vi "Initialize Core.vi"(8 "error in":errorcluster, 10 "Shared Resources":refnum<class "Shared Resources.lvclass">, 11 "Tx Acyclic Labels Execution Unit in":refnum<class "Tx Acyclic Labels Execution Unit.lvclass">) -> (0 "error out":errorcluster, 3 "Tx Acyclic Labels Execution Unit out":refnum<class "Tx Acyclic Labels Execution Unit.lvclass">)   [LabVIEW 2020, in "AIM ARINC 429 Engine.lvlib" / "Implementation.lvlib" / "Tx Acyclic Labels Execution Unit.lvclass"]
uses:
  Tx Acyclic Labels Execution Unit.lvclass
  C:/git/ni/niveristand-aim-arinc429-custom-device/Source/Custom Device Support/Engine/Implementation/Execution Unit/Execution Unit.lvclass
  Shared Resources/Shared Resources.lvclass
  Execution Unit/Execution Unit.lvclass/Execution Unit.ctl
  Tx Acyclic Labels Execution Unit.lvclass/Tx Acyclic Labels Execution Unit.ctl
  Execution Unit/Read board handle.vi
  Hardware API/AIM ARINC 429 Hardware API.lvlib
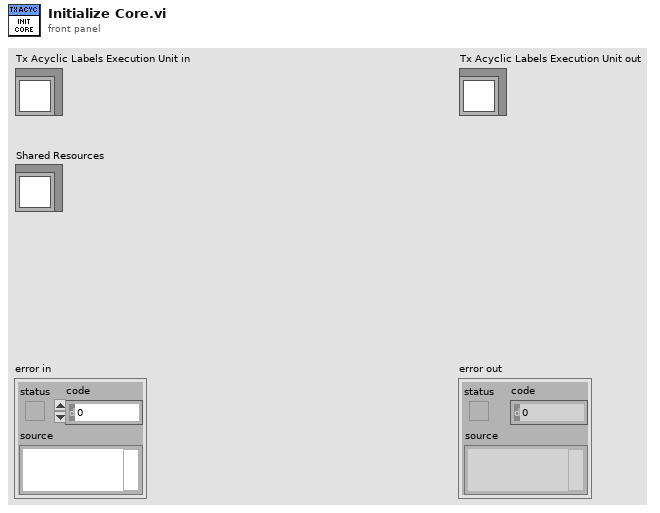
[diagram p1: front panel]
types:
  T1 = typedef "RT Hardware Channel Settings.ctl" = cluster{"channel #":u16, "channel handle":u64, "labels settings for RT":T2[], "speed":T10}
  T2 = typedef "RT Label Settings.ctl" = cluster{"Name":string, "xmlName":string, "label":T3, "transfer period":u32, "SDI_Enabled":bool, "SDI":u8, "parameter driver data":T4, "transfer type":T8, "has timestamp?":bool, "Label Disable/Trigger Channel Reference":T7, "Message Handle":u64, "Initialized?":bool, "Word Initial Raw Value":u32, "Label Timestamp Channel Data Reference":T9, "disabled":bool}
  T3 = typedef "Label.ctl" = u8
  T4 = typedef "RT Parameters.ctl" = cluster{"parameter definitions":T5[], "Tx parameter refs":T7[]}
  T5 = typedef "Parameter Definition.ctl" = cluster{"start index":i32, "size":i32, "encoding":T6, "signed":bool, "scale multiplier":dbl, "scale offset":dbl, "default value":dbl}
  T6 = typedef "Encoding and Decoding.lvlib/Encoding.ctl" = enum16{"BNR", "BCD", "Discrete"}
  T7 = typedef "Custom Device API.lvlib/Custom Device Item Ref.ctl" = u64
  T8 = typedef "Transfer Type.ctl" = enum16{"Scheduled", "Acyclic", "Block", "Strobe"}
  T9 = typedef "Custom Device API.lvlib/Data Reference.ctl" = i32
  T10 = typedef "Transfer Speed.ctl" = enum16{"LO (12.5 kb/s)", "HI (100 kb/s)"}
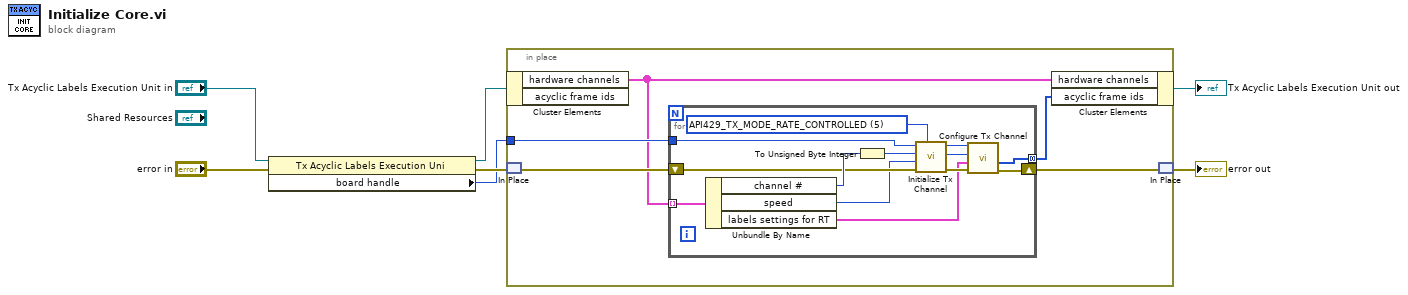
[diagram p0: block diagram]
diagram:
  n1 = property class="Tx Acyclic Labels Execution Uni"(reference="Tx Acyclic Labels Execution Unit in", error in="error in") -> (reference out=w6:refnum<class "Tx Acyclic Labels Execution Unit.lvclass">, error out=w7:errorcluster, "board handle"=w5:u8)
  n2 = in-place {
    in-place-border: w5 -> [w10]
    n3 = in-place-cluster #1(w6) -> ("hardware channels"=w9:T1[])  [unwired: 1 out]
    n4 = in-place-match #2(w7) -> (w12:errorcluster)
    n5 = for {
      tunnel: w9 -> [w19] mode=indexing
      tunnel: w10 -> [w23]
      tunnel: [w15] -> w8 mode=concatenating
      shift-right: [w16] -> w11
      shift-left: w12 -> [w24]
      w21 = u32 5 items=["API429_TX_MODE_FRAMING", "API429_TX_MODE_LOOP", "API429_TX_MODE_PHYS_REPLAY", "API429_TX_MODE_FRAMING_DYNTAG", "API429_TX_MODE_FIFO", "API429_TX_MODE_RATE_CONTROLLED"] ("mode")
      n6 = Unbundle By Name(w19) -> ("channel #"=w25:u16, "speed"=w13:T10, "labels settings for RT"=w14:T2[])
      n7 = To Unsigned Byte Integer(number=w25) -> (unsigned 8bit integer=w22:u8)
      n8 = call "Initialize Tx Channel.vi"("mode"=w21, "error in"=w24, "channel speed"=w13, "channel number"=w22, "board handle"=w23) -> ("error out"=w20:errorcluster, "channel number out"=w18:u8, "board handle out"=w17:u8)  [unwired: 4 in]
      n9 = call "Configure Tx Channel.vi"("error in"=w20, "labels settings for RT"=w14, "channel number in"=w18, "board handle in"=w17) -> ("error out"=w16:errorcluster, "acyclic frame ids out"=w15:u32[])  [unwired: 4 in, 2 out]
    }
    n10 = in-place-cluster #1("hardware channels"=w9, "acyclic frame ids"=w8) -> (→"Tx Acyclic Labels Execution Unit out":refnum<class "Tx Acyclic Labels Execution Unit.lvclass">)
    n11 = in-place-match #2(w11) -> (→"error out":errorcluster)
  }
